vi "pdw to raw PDW.vi"(0 "PDWs":T1[](array[typedef]), 5 "Fs fpGa":dbl, 7 "SPC":i32=1, 9 "gen for DF":bool, 11 "erorr in":errorcluster) -> (4 "Array":u64[][](array[numeric]), 6 "lfm lost":bool, 15 "erorr out":errorcluster)   [LabVIEW 2021]
uses:
  PDW_lv2.ctl
  mode_type.ctl
  pdw.ctl
panel:
  out "mod too wide":bool
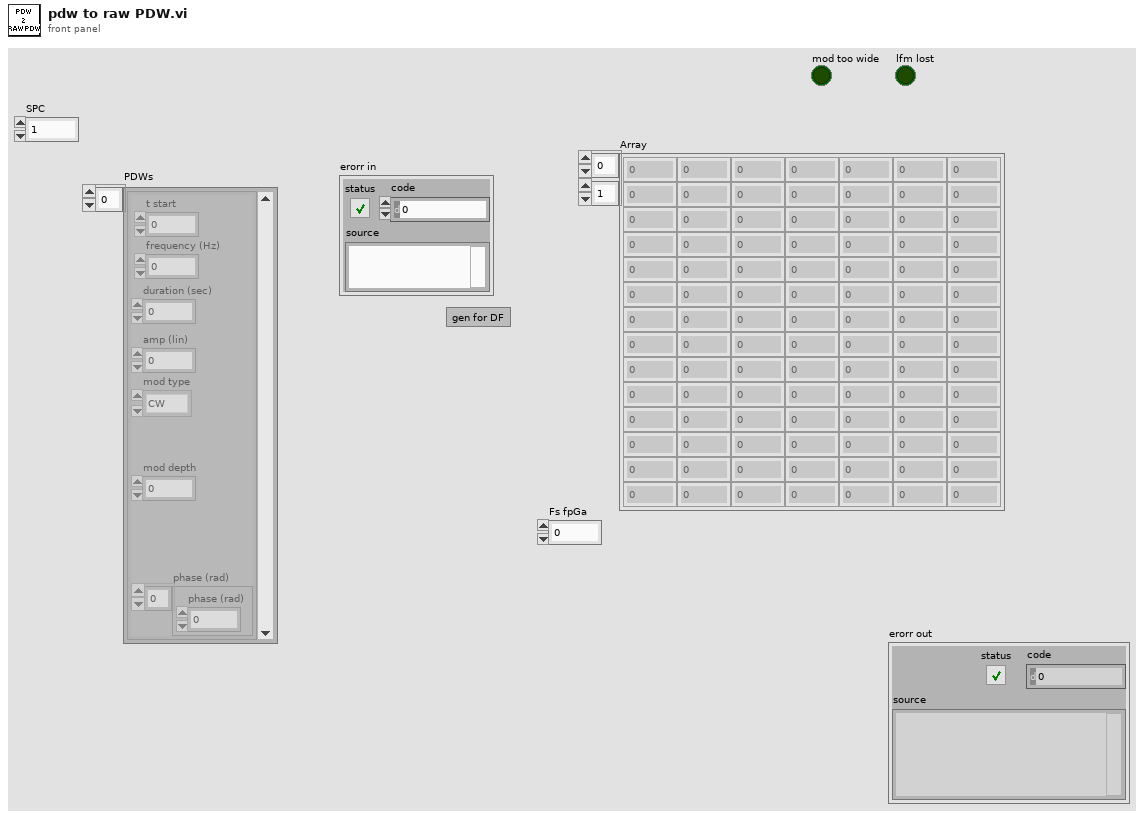
[diagram p1: front panel]
types:
  T1 = typedef "PDW_lv2.ctl" = cluster{"t start":dbl, "frequency (Hz)":dbl, "duration (sec)":dbl, "amp (lin)":dbl, "mod type":T2, "mod depth":dbl, "phase (rad)":dbl[]}
  T2 = typedef "mode_type.ctl" = enum8{"CW", "NC - CW", "NC - cw", "LFM", "BPSK", "QPSK"}
  T3 = typedef "pdw.ctl" = cluster{"PW":u32, "frequency shift":fxp<+/-,48,0>, "amp":fxp<+/-,18,1>, "mode type":T2, "mode depth":u32, "mode filter":u8, "phase shift":fxp<+/-,16,1>, "pulse shape filter":u8}
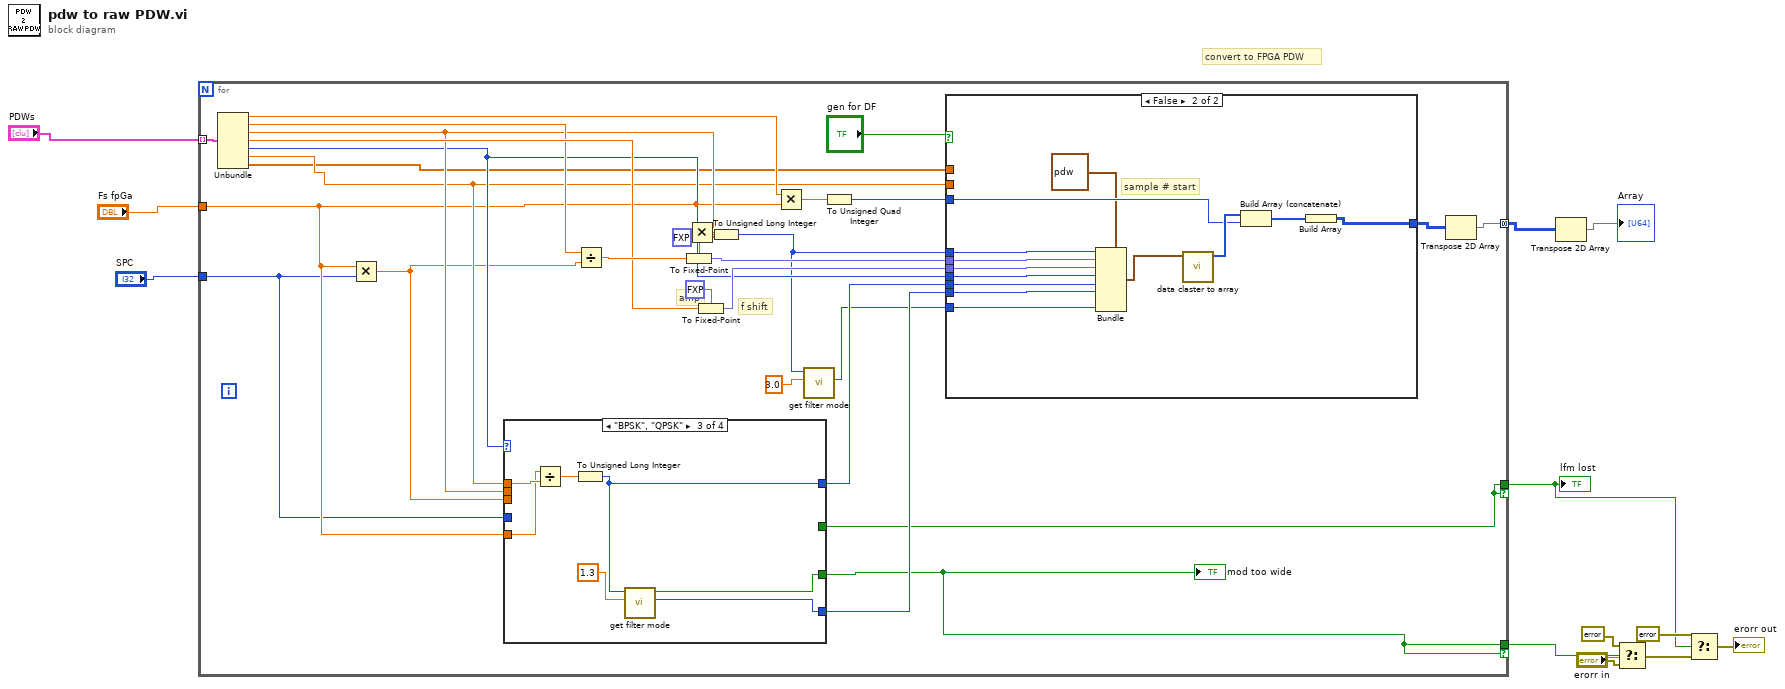
[diagram p0: block diagram]
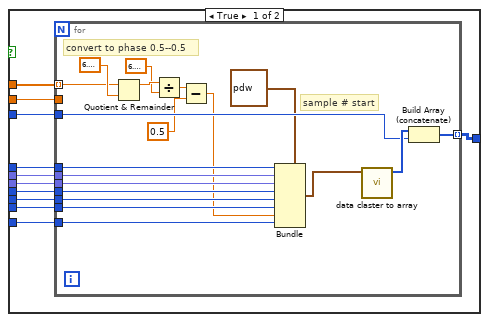
[diagram p2: hidden frame]
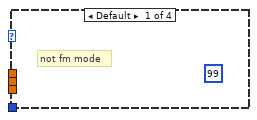
[diagram p3: hidden frame]
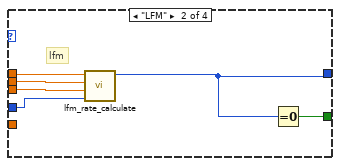
[diagram p4: hidden frame]
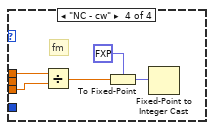
[diagram p5: hidden frame]
diagram:
  # "convert to FPGA PDW"
  n1 = for {
    tunnel: "PDWs" -> [w41] mode=indexing
    tunnel: [w22] -> w4 mode=concatenating
    tunnel: "Fs fpGa" -> [w17]
    tunnel: [w19] -> w2 if=w19
    tunnel: [w25] -> w8 if=w25
    tunnel: "SPC" -> [w16]
    # "amp"
    # "f shift"
    n2 = Unbundle(w41) -> ("t start"=w40:dbl, "frequency (Hz)"=w30:dbl, "duration (sec)"=w29:dbl, "amp (lin)"=w34:dbl, "mod type"=w28:T2, "mod depth"=w21:dbl, "phase (rad)"=w20:dbl[])
    n3 = Multiply(x=w17, y=w16) -> (x*y=w18:dbl)
    n4 = case shown="\"BPSK\", \"QPSK\"" w28 {
      tunnel: [_ w87 w94 _] -> w27
      tunnel: w18 -> [_ w90 _ w101]
      tunnel: w21 -> [_ w88 w97 w102]
      tunnel: w29 -> [_ w89 _ _]
      tunnel: [_ _ w95 _] -> w26
      tunnel: [_ _ w93 _] -> w25
      tunnel: [_ w86 _ _] -> w19
      tunnel: w17 -> [_ _ w92 _]
      tunnel: w16 -> [_ w85 _ _]
      frame Default {
        (unwired) u32 99 ("integer (fxp cast)")
        # "not fm mode"
      }
      frame "LFM" {
        # "lfm"
        n5 = call "lfm_rate_calculate.vi"("SPC"=w85, "fs"=w90, "pw"=w89, "f span"=w88) -> ("integer (fxp cast)"=w87:u32)  [unwired: 7 in]
        n6 = Equal To 0?(x=w87) -> (x = 0?=w86:bool)
      }
      frame "BPSK", "QPSK" {
        n7 = Divide(x=w92, y=w97) -> (x/y=w96:dbl)
        n8 = To Unsigned Long Integer(number=w96) -> (unsigned 32bit integer=w94:u32)
        n9 = call "get filter mode.vi"("filter rate"=1.3 ("y"), "Numeric in"=w94) -> ("filter mode"=w95:i32, "no fit filter"=w93:bool)  [unwired: 8 in]
      }
      frame "NC - cw" {
        # "fm"
        n10 = Divide(x=w102, y=w101) -> (x/y=w98:dbl)
        n11 = To Fixed-Point(fixed-point type=fxp<+,32,-16> 0.0, number=w98) -> (fixed-point=w100:fxp<+,32,-16>)
        n12 = Fixed-Point to Integer Cast(1:w100) -> ()  [unwired: 1 out]
      }
    }
    "mod too wide" <- w25
    n13 = Divide(x=w30, y=w18) -> (x/y=w38:dbl)
    n14 = To Fixed-Point(fixed-point type=fxp<+/-,48,0> 0.0 ("frequency shift"), number=w38) -> (fixed-point=w36:fxp<+/-,48,0>)
    n15 = Multiply(x=w29, y=w17) -> (x*y=w35:dbl)
    n16 = To Fixed-Point(fixed-point type=fxp<+/-,18,1> 0.0 ("I"), number=w34) -> (fixed-point=w32:fxp<+/-,18,1>)
    n17 = To Unsigned Long Integer(number=w35) -> (unsigned 32bit integer=w15:u32)
    n18 = Multiply(x=w40, y=w17) -> (x*y=w39:dbl)
    n19 = call "get filter mode.vi"("filter rate"=3.0, "Numeric in"=w15) -> ("filter mode"=w13:i32)  [unwired: 8 in, 1 out]
    n20 = To Unsigned Quad Integer(1:w39) -> (0:w31:u64)
    n21 = case shown="False" "gen for DF" {
      tunnel: w36 -> [w52 w84]
      tunnel: w32 -> [w51 w83]
      tunnel: w31 -> [w50 w81]
      tunnel: [w49 w74] -> w23
      tunnel: w15 -> [w48 w78]
      tunnel: w28 -> [w47 w77]
      tunnel: w27 -> [w46 w73]
      tunnel: w26 -> [w45 w76]
      tunnel: w21 -> [w44 _]
      tunnel: w20 -> [w43 _]
      tunnel: w13 -> [w42 w72]
      frame True {
        n22 = for {
          tunnel: w52 -> [w71]
          tunnel: w51 -> [w70]
          tunnel: w50 -> [w68]
          tunnel: [w65] -> w49 mode=indexing
          tunnel: w48 -> [w64]
          tunnel: w47 -> [w63]
          tunnel: w46 -> [w62]
          tunnel: w45 -> [w61]
          tunnel: w44 -> [_]
          tunnel: w43 -> [w54] mode=indexing
          tunnel: w42 -> [w53]
          # "convert to phase 0.5--0.5"
          # "sample # start"
          n23 = Quotient & Remainder(x=w54, y=6.283185307179586) -> (x-y*floor(x/y)=w59:dbl)  [unwired: 1 out]
          n24 = Divide(x=w59, y=6.283185307179586) -> (x/y=w57:dbl)
          n25 = Subtract(x=w57, y=0.5) -> (x-y=w55:dbl)
          n26 = Bundle(cluster=T3 {"PW"=0, "frequency shift"=0.0, "amp"=0.0, "mode type"=enum."CW", "mode depth"=0, "mode filter"=0, "phase shift"=0.0, "pulse shape filter"=0} ("Cluster"), "PW"=w64, "frequency shift"=w71, "amp"=w70, "mode type"=w63, "mode depth"=w62, "mode filter"=w61, "phase shift"=w55, "pulse shape filter"=w53) -> (w66:T3)
          n27 = call "data claster to array.vi"("Cluster"=w66) -> ("Array"=w69:u64[])  [unwired: 10 in]
          n28 = Build Array (concatenate)(w69, w68) -> (w65:u64[])
        }
      }
      frame False {
        # "sample # start"
        n29 = Bundle(cluster=T3 {"PW"=0, "frequency shift"=0.0, "amp"=0.0, "mode type"=enum."CW", "mode depth"=0, "mode filter"=0, "phase shift"=0.0, "pulse shape filter"=0} ("Cluster"), "PW"=w78, "frequency shift"=w84, "amp"=w83, "mode type"=w77, "mode depth"=w73, "mode filter"=w76, "pulse shape filter"=w72) -> (w79:T3)  [unwired: 1 in]
        n30 = call "data claster to array.vi"("Cluster"=w79) -> ("Array"=w82:u64[])  [unwired: 10 in]
        n31 = Build Array (concatenate)(w82, w81) -> (w75:u64[])
        n32 = Build Array(w75) -> (w74:u64[][])
      }
    }
    n33 = Transpose 2D Array(2D array=w23) -> (transposed array=w22:u64[][])
  }
  "lfm lost" <- w2
  n34 = Transpose 2D Array(2D array=w4) -> (transposed array=→"Array":u64[][])
  n35 = Select(t=errorcluster {"status"=TRUE, "code"=5432, "source"="PSK mod too wide"} ("error out"), s=w8, f="erorr in") -> (s? t:f=w6:errorcluster)
  n36 = Select(t=errorcluster {"status"=TRUE, "code"=5432, "source"="The LFM value lost, pls take higher value for it"} ("error out"), s=w2, f=w6) -> (s? t:f=→"erorr out":errorcluster)
